vi "ReadFile.vi"(8 "error in (no error)":errorcluster, 10 "ExpData File Path":path, 11 "ExpData In":refnum<class "ExpData.lvclass">) -> (0 "error out":errorcluster, 1 "Marked":bool, 2 "MetaData":string, 3 "ExpData Out":refnum<class "ExpData.lvclass">)   [LabVIEW 2016, in "ExpData.lvclass"]
uses:
  ExpData.lvclass
  typedef/ColHeader.ctl
  ExpData.lvclass/ExpData.ctl
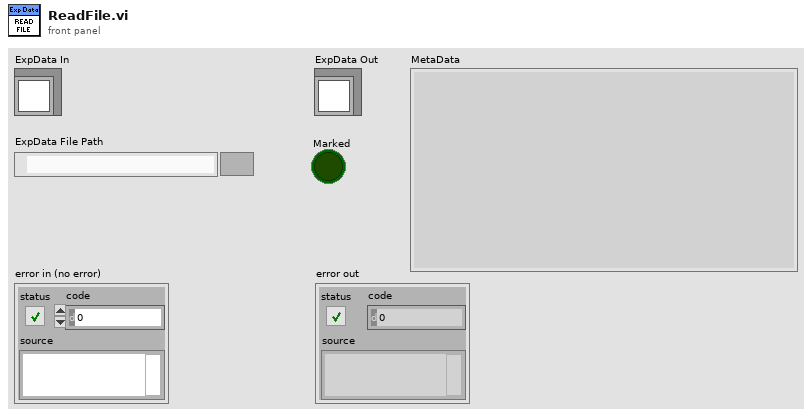
[diagram p1: front panel]
types:
  T1 = typedef "ExpData.lvclass/ColHeader.ctl" = cluster{"Name":string, "Index":i32, "Size":i32}
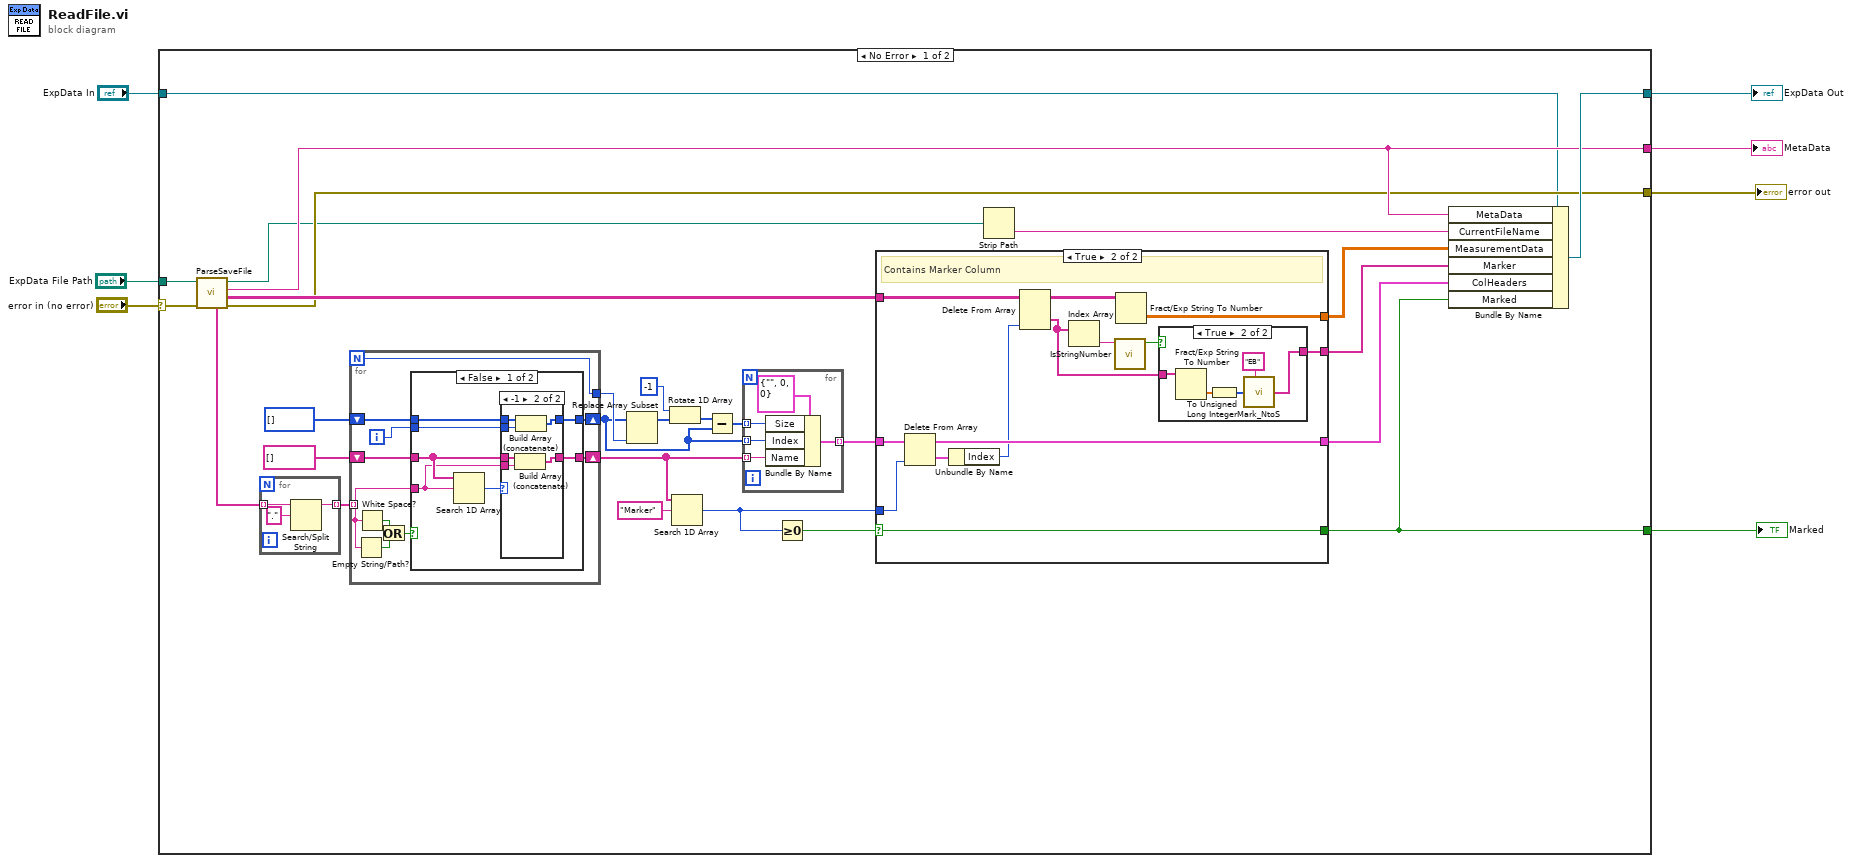
[diagram p0: block diagram]
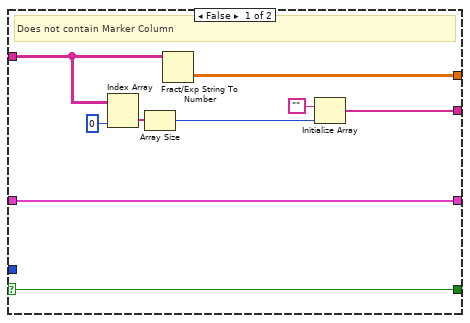
[diagram p4: hidden frame]
diagram:
  n1 = case shown="No Error" "error in (no error)" {
    selector: "error in (no error)" -> [w30 w100]
    tunnel: "ExpData File Path" -> [w31 _]
    tunnel: "ExpData In" -> [w8 w99]
    tunnel: [w32 w99] -> w4
    tunnel: [w10 w100] -> w3
    tunnel: [w16 _] -> w2
    tunnel: [w12 _] -> w1
    frame No Error {
      n2 = call "ParseSaveFile.vi"("error in (no error)"=w30, "ExpData File Path"=w31) -> ("error out"=w10:errorcluster, "Data"=w11:string[][], "MetaData"=w12:string, "dup path"=w9:path, "Column Headers"=w13:string[])  [unwired: 5 in]
      n3 = for {
        tunnel: w13 -> [w98] mode=indexing
        tunnel: [w96] -> w29 mode=indexing
        n4 = Search/Split String(string=w98, search string/char (-)=".") -> (substring before match=w96:string)  [unwired: 1 in, 2 out]
      }
      n5 = for {
        N -> [w45]
        tunnel: w29 -> [w44] mode=indexing
        shift-right: [w48] -> w17
        shift-left: string[] [] -> [w49]
        shift-right: [w46] -> w22
        shift-left: i32[] [] -> [w47]
        tunnel: [w45] -> w26
        i -> [w50]
        n6 = Empty String/Path?(string/path=w44) -> (empty?=w41:bool)
        n7 = White Space?(1:w44) -> (0:w42:bool)
        n8 = Or(x=w42, y=w41) -> (x .or. y?=w43:bool)
        n9 = case shown="False" w43 {
          tunnel: w50 -> [w56 _]
          tunnel: w49 -> [w55 w66]
          tunnel: [w54 w66] -> w48
          tunnel: w47 -> [w53 w67]
          tunnel: [w52 w67] -> w46
          tunnel: w44 -> [w51 _]
          frame False {
            n10 = Search 1D Array(1D array=w55, element=w51) -> (index of element=w57:i32)  [unwired: 1 in]
            n11 = case shown="-1" w57 {
              tunnel: w51 -> [_ w65]
              tunnel: w56 -> [_ w60]
              tunnel: w55 -> [w58 w64]
              tunnel: [w58 w63] -> w54
              tunnel: w53 -> [w59 w62]
              tunnel: [w59 w61] -> w52
              frame Default {
              }
              frame -1 {
                n12 = Build Array (concatenate)(w64, w65) -> (w63:string[])
                n13 = Build Array (concatenate)(w62, w60) -> (w61:i32[])
              }
            }
          }
          frame True {
          }
        }
      }
      n14 = Replace Array Subset(array=w22, new element=w26) -> (w25:i32[])  [unwired: 1 in]
      n15 = Rotate 1D Array(1:w25, 2:-1 ("n")) -> (0:w24:i32[])
      n16 = Search 1D Array(1D array=w17, element="Marker") -> (index of element=w34:i32)  [unwired: 1 in]
      n17 = Subtract(x=w24, y=w22) -> (x-y=w23:i32[])
      n18 = for {
        tunnel: w23 -> [w40] mode=indexing
        tunnel: w22 -> [w39] mode=indexing
        tunnel: w17 -> [w38] mode=indexing
        tunnel: [w37] -> w21 mode=indexing
        n19 = Bundle By Name(cluster=T1 {"Name"="", "Index"=0, "Size"=0} ("ColHeader"), "Size"=w40, "Index"=w39, "Name"=w38) -> (w37:T1)
      }
      n20 = Greater Or Equal To 0?(x=w34) -> (x >= 0?=w18:bool)
      n21 = case shown="True" w18 {
        selector: w18 -> [w68 w88]
        tunnel: w21 -> [w73 w83]
        tunnel: w34 -> [_ w81]
        tunnel: w11 -> [w70 w87]
        tunnel: [w76 w89] -> w15
        tunnel: [w73 w82] -> w14
        tunnel: [w74 w86] -> w33
        tunnel: [w68 w88] -> w16
        frame False {
          # "Does not contain Marker Column"
          n22 = Index Array(array=w70, index (col)=0 ("disabled index (col)")) -> (element=w71:string[])  [unwired: 1 in]
          n23 = Array Size(array=w71) -> (size(s)=w69:i32)
          n24 = Fract/Exp String To Number(string=w70) -> (number=w74:dbl[][])  [unwired: 3 in, 1 out]
          n25 = Initialize Array("", w69) -> (w76:string[])
        }
        frame True {
          # "Contains Marker Column"
          n26 = Delete From Array(array=w83, index=w81) -> (deleted portion=w78:T1, array with subset deleted=w82:T1[])  [unwired: 1 in]
          n27 = Unbundle By Name(w78) -> ("Index"=w77:i32)
          n28 = Delete From Array(array=w87, index (col)=w77) -> (deleted portion=w79:string[], array with subset deleted=w80:string[][])  [unwired: 2 in]
          n29 = Index Array(array=w79) -> (element=w85:string)  [unwired: 1 in]
          n30 = call "IsStringNumber.vi"("String"=w85) -> ("Start with Number"=w84:bool)  [unwired: 7 in, 3 out]
          n31 = Fract/Exp String To Number(string=w80) -> (number=w86:dbl[][])  [unwired: 3 in, 1 out]
          n32 = case shown="True" w84 {
            tunnel: [w90 w94] -> w89
            tunnel: w79 -> [w90 w93]
            frame False {
            }
            frame True {
              n33 = Fract/Exp String To Number(string=w93) -> (number=w92:dbl[])  [unwired: 3 in, 1 out]
              n34 = To Unsigned Long Integer(number=w92) -> (unsigned 32bit integer=w95:u32[])
              n35 = call "Mark_NtoS.vi"("Marker(Low->High)"="EB", "MarkerNumber"=w95) -> ("MarkerString"=w94:string[])  [unwired: 3 in]
            }
          }
        }
      }
      n36 = Strip Path(path=w9) -> (name=w19:string)  [unwired: 1 out]
      n37 = Bundle By Name(cluster=w8, "MetaData"=w12, "CurrentFileName"=w19, "MeasurementData"=w33, "Marker"=w15, "ColHeaders"=w14, "Marked"=w16) -> (w32:refnum<class "ExpData.lvclass">)
    }
    frame Error {
    }
  }
  "ExpData Out" <- w4
  "error out" <- w3
  "Marked" <- w2
  "MetaData" <- w1
